vi "Get date and time in seconds sequential.vi"(2 "error in (no error)":errorcluster) -> (0 "error out":errorcluster, 1 "current time":timestamp)   [LabVIEW 2020]
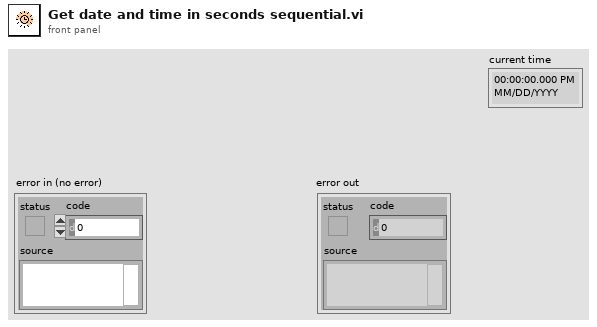
[diagram p1: front panel]
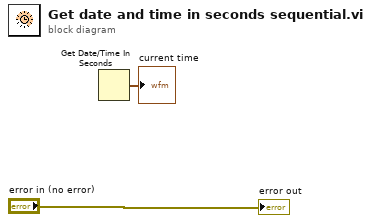
[diagram p0: block diagram]
diagram:
  n1 = Get Date/Time In Seconds() -> (seconds since 1Jan1904=→"current time":timestamp)
  "error out" <- "error in (no error)"
